vi "FPGA.vi"() -> ()   [LabVIEW 2020]
uses:
  <vilib>/Platform/TimedLoop/XDataNode/timing_clust.ctl
  <vilib>/Platform/TimedLoop/XDataNode/nitl_modes.ctl
  <vilib>/Platform/TimedLoop/XDataNode/wakeup.ctl
  <vilib>/rvi/Analysis/measure/FFT/simModelSupport/niFPGA FFT Sim Properties.ctl
  <vilib>/rvi/Analysis/measure/FFT/simModelSupport/niFPGA FFT Sim Types.ctl
  <vilib>/rvi/Analysis/measure/FFT/simModelSupport/niFpgaFFTSimArithmeticProperties.ctl
  <vilib>/rvi/Analysis/measure/FFT/simModelSupport/niFpgaFFTSimDfxp.ctl
  <vilib>/fxp/LVFixedPointQuantizationPolicyTypeDef.ctl
  <vilib>/rvi/eio/common/nirviEmuTemplateMethod_errors.vi
  <vilib>/rvi/DataTransferAndStorage/Container/Common/niFpgaContainerGetUniqueNameForEmu.vi
  <vilib>/rvi/DataTransferAndStorage/Container/Common/niFpgaContainerSetEmuInfo.vi
  <vilib>/rvi/eio/common/nirviEmuReportErrorAndStop.vi
  <vilib>/rvi/DataTransferAndStorage/Container/Common/niFpgaContainerExecOnDevCompGetState.vi
  <vilib>/rvi/Emulation/niFpgaEmulationIsFPGAContextNoSignature.vi
  <vilib>/rvi/Emulation/niFpgaSctlEmulationGetInTimedLoop.vi
  <vilib>/rvi/errors/niFpgaSetErrorForExecOnDevCompSimple.vi
  <vilib>/rvi/FIFO/Fifo_Resource/nirvififoEmulationSetSize.vi
  <vilib>/rvi/FIFO/Fifo_Resource/nirviFifoEmulationQueueMgr.vi
  <instcachedir>/0/nirviFifoEmulationQueueMgr_E5CAEC123FF24DC58D834DCA3CDAA9B5.lvgen/nirviFifoEmulationQueueMgr_E5CAEC123FF24DC58D834DCA3CDAA9B5_003.vi
  <vilib>/rvi/FIFO/Fifo_Resource/nirvififoEmulationDetermineInputValidOut.vi
  <vilib>/rvi/FIFO/Fifo_Resource/nirvififoEmulationCreateLock.vi
  <vilib>/rvi/Emulation/niFpgaProcessEmulError.vi
  <vilib>/rvi/FIFO/Fifo_Resource/nirvififoEmulationObtainLock.vi
  <vilib>/rvi/FIFO/Fifo_Resource/nirvififoEmulationReleaseLock.vi
  <vilib>/rvi/occurrence/nirviWaitOnOccurrenceBase.vi
  <vilib>/rvi/errors/nirviReportUnexpectedCaseInternalError.vi
  <vilib>/rvi/errors/nirviReportUnexpectedCaseInternalError (U32).vi
  <vilib>/Utility/error.llb/Clear Errors.vi
  <vilib>/rvi/interface/RandomDataEmulation/niFpgaRandomDataHandleErrors.vi
  <vilib>/rvi/Emulation/niFpgaEmulationReportErrorSimple.vi
  <vilib>/rvi/Emulation/niFpgaGetClockAttributes.vi
  <vilib>/rvi/Emulation/niFpgaCriticalErrorInLSC.vi
  <vilib>/rvi/Analysis/measure/FFT/simModelSupport/niFpgaFFTSimModelCore.vi
  <vilib>/eio/EIONode/EIONode.xnode
  <vilib>/rvi/LocalResourceManager/LocalResourceManager.xnode
  <vilib>/rvi/DataTransferAndStorage/Container/XNode/niFpgaContainer.xnode
  <vilib>/rvi/FIFO/Fifo_Resource/niFpgaFifoEmulationRefIn.vi
  <vilib>/Platform/TimedLoop/XDataNode/XDataNode.xnode
  <vilib>/rvi/interface/RandomDataEmulation/nirviRandomDataFpgaReadWriteTemplate.vi
  <vilib>/rvi/Analysis/measure/FFT/XNode/niFpgaFFT.xnode
  <vilib>/rvi/FXPMathLib/FxpInterpret/XNode/nifxpmath_Interpret.xnode
  <vilib>/Platform/TimedLoop/XDataNode/XDNodeRunTimeDep.lvlib
panel:
  out "Timed Out? FIFO out index 2":bool
  out "Timed Out? FIFO out IMG 2":bool
  out "Timed Out? FIFO out REAL 2":bool
  out "sort time (us)":u32
  out "Timed Out? FIFO in IMG":bool
  out "Timed Out? FIFO in REAL":bool
  out "Timed Out? FIFO out REAL":bool
  out "Timed Out? FIFO out IMG":bool
  out "Timed Out? FIFO out index":bool
  in  "FFT loop iterations":i32
  in  "auto stop":bool
  out "FFT time (uSec)":u32
  out "data collection time (uSec)":u32
  in  "Loop number":i32
  out "Element":fxp<+/-,24,7>
  out "Actual loop rate":u32
  in  "Rate (uSec)":u32 caption="Count(uSec)"
  out "Timed Out?":bool
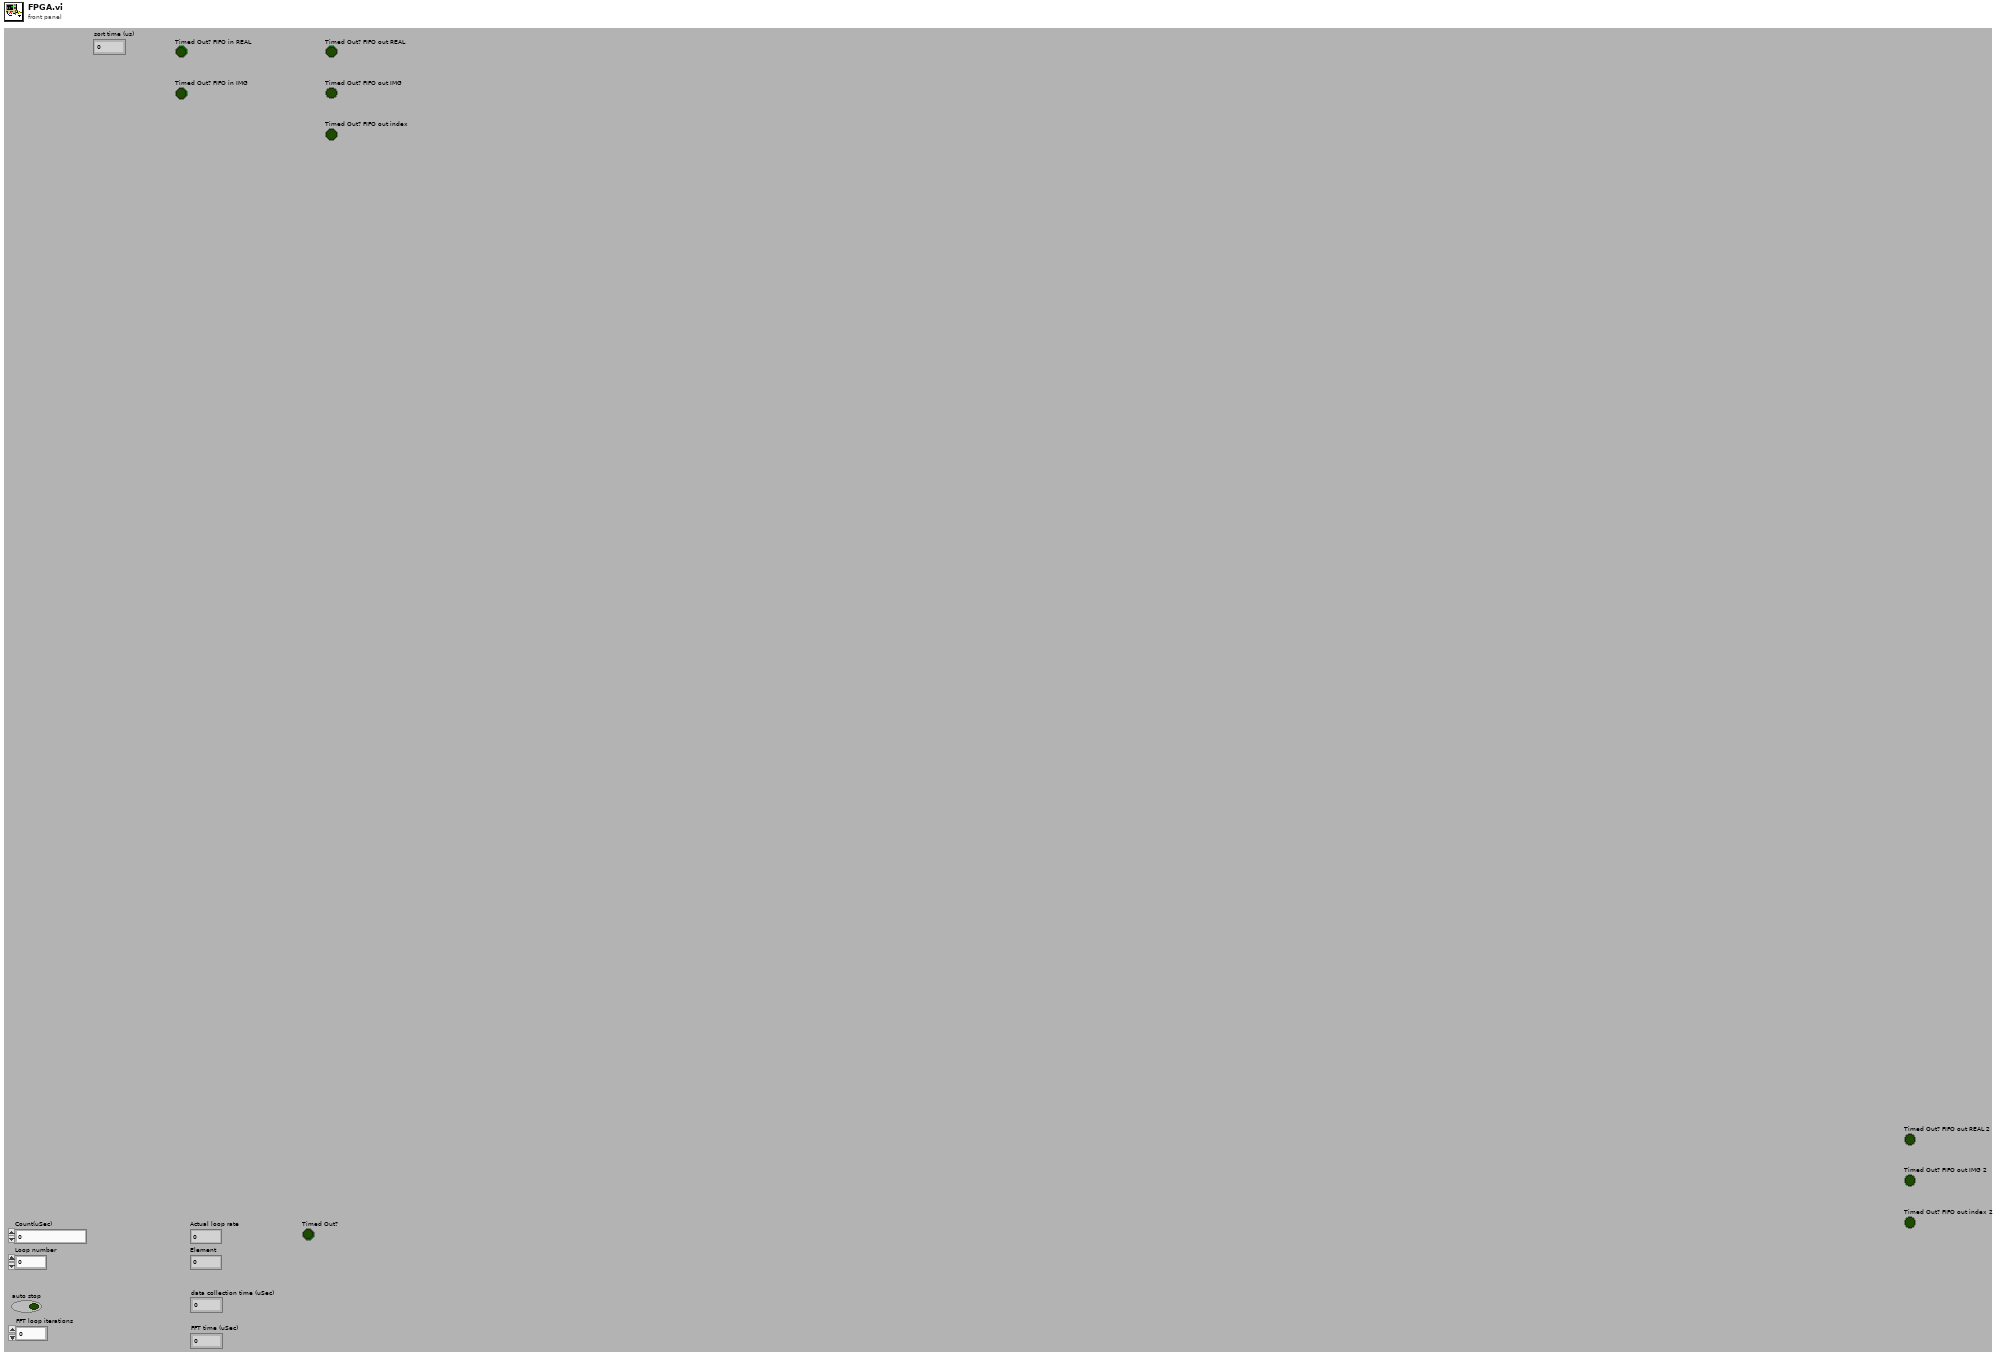
[diagram p1: front panel]
types:
  T1 = typedef "XDNodeRunTimeDep.lvlib/timing_clust.ctl" = cluster{"Expected End [f-1]":u64, "Actual End [f-1]":u64, "Finished Late? [f-1]":bool, "Expected End [i-1]":u64, "Actual End [i-1]":u64, "Finished Late? [i-1]":bool, "Expected Start [i]":u64, "Actual Start [i]":u64, "Expected Start [f]":u64, "Actual Start [f]":u64, "Source Name":string, "Structure Name":string, "Period":i64, "Deadline":i64, "Offset":i64, "Start":i64, "Priority":i32, "Timeout":i32, "Mode":T2, "Wakeup Reason":T3, "Error":errorcluster, "Source Type":string, "Secondary Source Type":string, "Global End Time":u64, "Global Start Time":u64, "Frame Duration":u64, "Iteration Duration":u64, "Assigned CPU":i32, "I/O Scan Engine Mode":u32}
  T2 = typedef "XDNodeRunTimeDep.lvlib/nitl_modes.ctl" = enum32{"No Change", "Process missed periods, maintain original phase", "Discard missed periods, maintain original phase", "Process missed periods, ignore original phase", "Discard missed periods, ignore original phase"}
  T3 = typedef "XDNodeRunTimeDep.lvlib/wakeup.ctl" = enum32{"Normal", "Aborted", "Asynchronous wakeup", "Timing source error", "Timed loop error", "Timeout"}
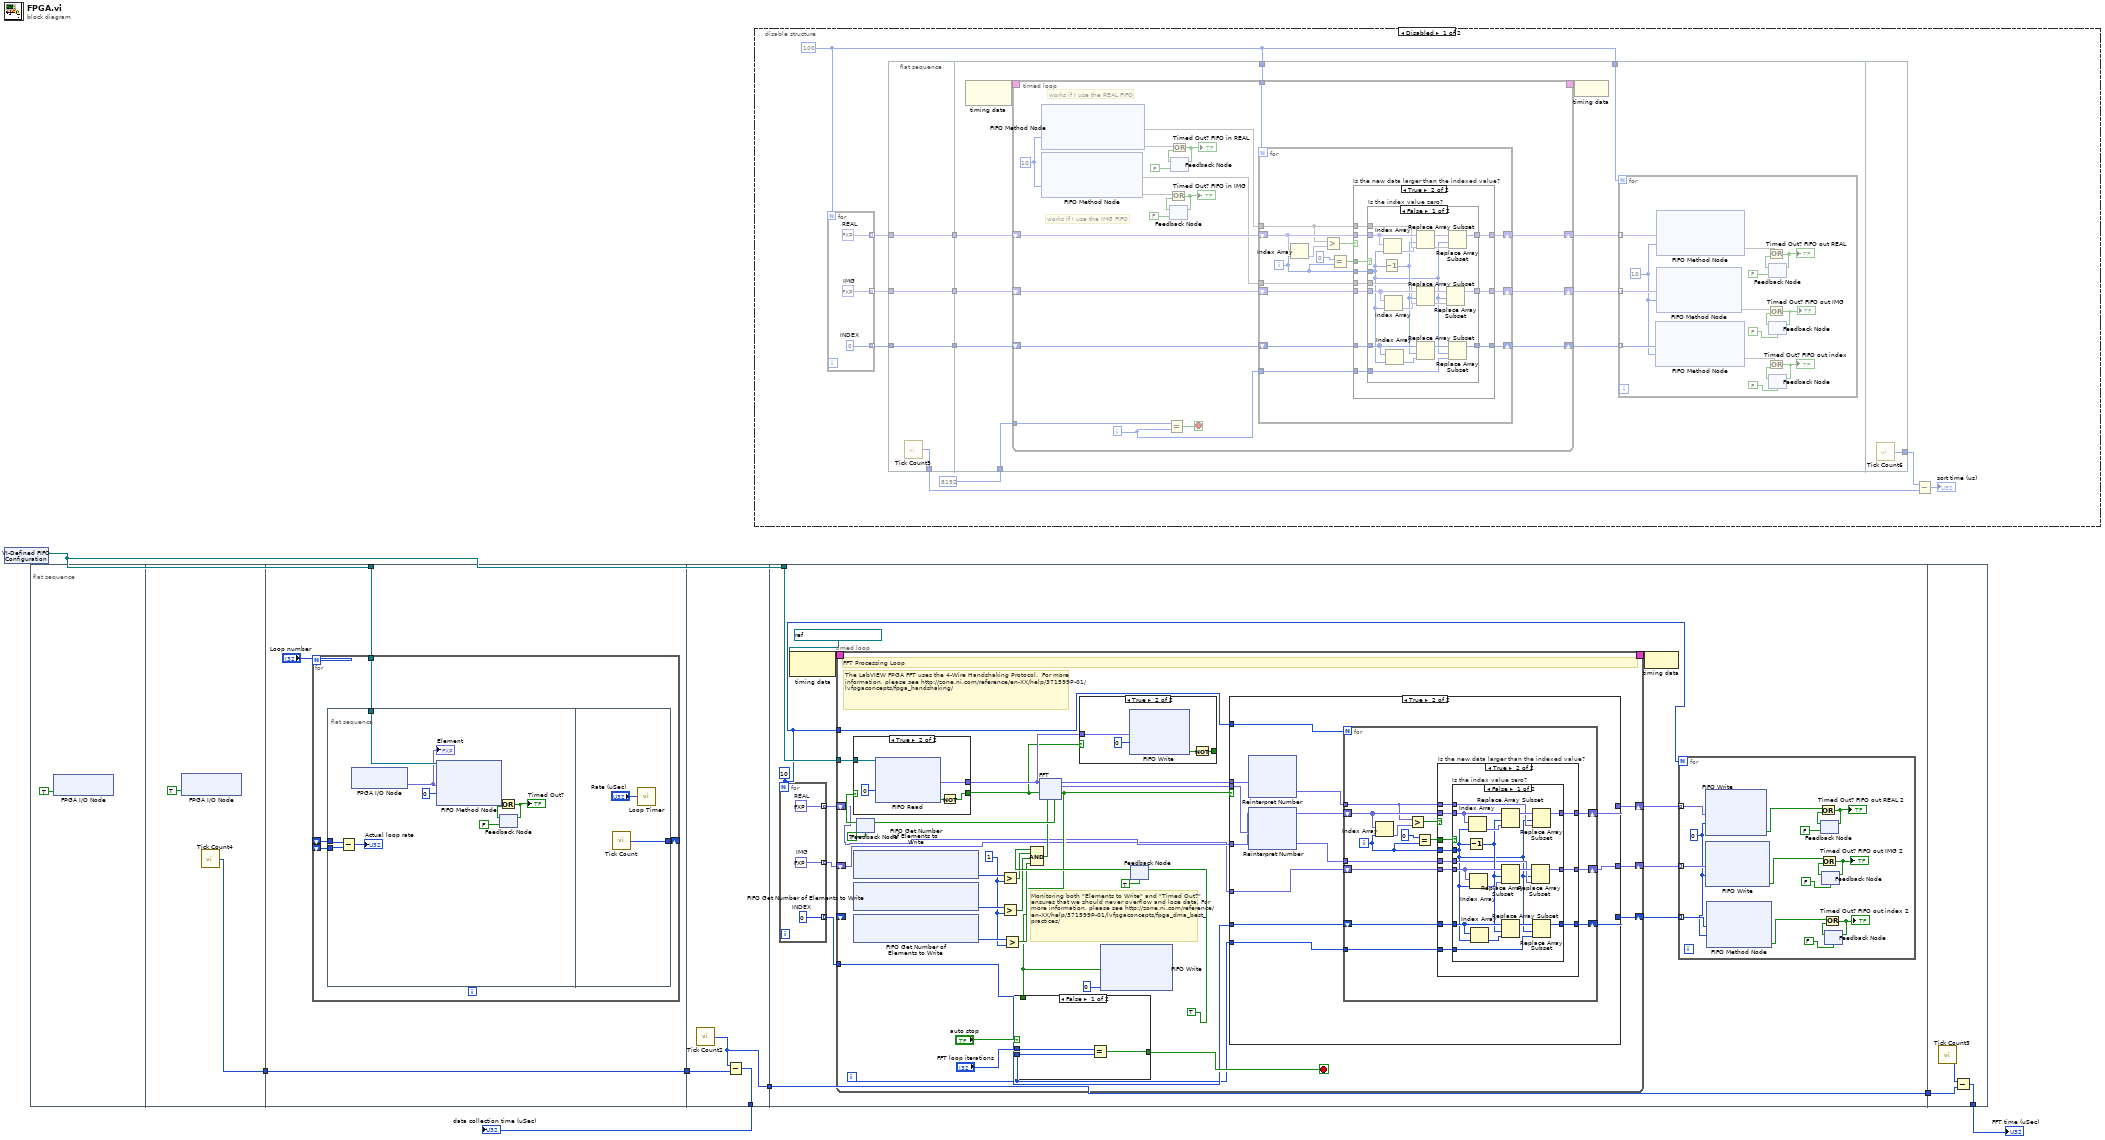
[diagram p0: block diagram]
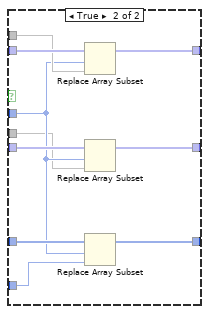
[diagram p3: hidden frame]
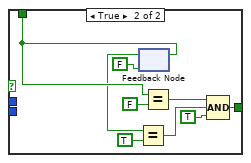
[diagram p5: hidden frame]
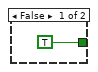
[diagram p6: hidden frame]
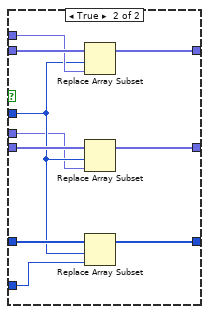
[diagram p9: hidden frame]
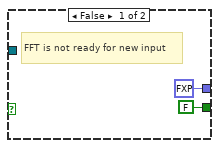
[diagram p10: hidden frame]
diagram:
  n1 = xnode "VI-Defined FIFO Configuration"() -> ("FIFO Out"=w7:refnum<k21>)
  n2 = flat-sequence {
    tunnel: [w9] -> w6
    tunnel: w7 -> [w13]
    tunnel: w6 -> [w11]
    tunnel: [w11] -> w5
    tunnel: w5 -> [w32]
    tunnel: [w31] -> w4
    tunnel: [w30] -> w3
    tunnel: w7 -> [w42]
    tunnel: w3 -> [w41]
    tunnel: [w41] -> w2
    tunnel: w2 -> [w223]
    tunnel: [w222] -> w1
    frame #0 {
      n3 = xnode "FPGA I/O Node"("Mod1/Stop"=TRUE) -> ()  [unwired: 1 in, 1 out]
    }
    frame #1 {
      n4 = xnode "FPGA I/O Node"("Mod1/Start"=TRUE) -> ()  [unwired: 1 in, 1 out]
      n5 = call "Tick Count4"() -> ("Tick Count(uSec)"=w9:u32)
    }
    frame #2 {
      n6 = for {
        N: "Loop number" -> [_]
        shift-right: [w17] -> _
        shift-left: _ -> [w16]
        shift-left: _ -> [w15]
        tunnel: w13 -> [w14]
        n7 = flat-sequence {
          tunnel: w16 -> [w27]
          tunnel: w15 -> [w26]
          tunnel: w14 -> [w19]
          tunnel: [w28] -> w17
          frame #0 {
            n8 = Subtract(x=w27, y=w26) -> (x-y=→"Actual loop rate":u32)
            n9 = xnode "FPGA I/O Node"() -> ("Mod1/AI0"=w18:fxp<+/-,24,7>)  [unwired: 1 in, 1 out]
            "Element" <- w18
            n10 = xnode ("FIFO Method Node")("Element"=w18, "Timeout"=0, "FIFO In"=w19) -> ("Timed Out?"=w23:bool)  [unwired: 1 in, 2 out]
            n11 = feedback #1(FALSE) -> (w22:bool)
            n12 = Or(x=w23, y=w22) -> (x .or. y?=w21:bool)
            "Timed Out?" <- w21
            n13 = feedback-in #1(w21) -> ()
          }
          frame #1 {
            n14 = call "Tick Count"() -> ("Tick Count(uSec)"=w28:u32)
            n15 = call "Loop Timer"("Count(uSec)"="Rate (uSec)") -> ()  [unwired: 1 out]
          }
        }
      }
    }
    frame #3 {
      n16 = call "Tick Count2"() -> ("Tick Count(uSec)"=w30:u32)
      n17 = Subtract(x=w30, y=w32) -> (x-y=w31:u32)
    }
    frame #4 {
      w34 = 10
      n18 = for {
        N: w34 -> [_]
        tunnel: [w63] -> w40 mode=indexing
        tunnel: [w62] -> w38 mode=indexing
        tunnel: [w61] -> w39 mode=indexing
        w61 = fxp<+/-,32,21> 0.0  # IMG
        w62 = 0  # INDEX
        w63 = fxp<+/-,32,21> 0.0  # REAL
      }
      n19 = node-c288(refnum<k21> "40 MHz Onboard Clock" ("Source Name")) -> (w44:T1)
      n20 = timed-loop {
        timing: w44 -> [_]
        timing-out: [_] -> w43
        tunnel: w42 -> [w92]
        tunnel: w38 -> [w70]
        tunnel: w34 -> [w64]
        shift-right: [w66] -> w35
        shift-left: _ -> [_]
        shift-right: [w67] -> w37
        shift-left: w39 -> [w71]
        shift-right: [w68] -> w36
        shift-left: w40 -> [w72]
        i -> [w69]
        stop <- w77 stop-if-true
        w86 = u32 1 ("y")
        # "Monitoring both \"Elements to Write\" and \"Timed Out?\" ensures that we should never overflow and lose data. For more information, please see http://zone.ni.com/reference/en-XX/help/371599P-01/lvfpgaconcepts/fpga_dma_best_practices/"
        # "The LabVIEW FPGA FFT uses the 4-Wire Handshaking Protocol.  For more information, please see http://zone.ni.com/reference/en-XX/help/371599P-01/lvfpgaconcepts/fpga_handshaking/"
        # "FFT Processing Loop"
        n21 = xnode ("FIFO Get Number of Elements to Write")() -> ("Number of Elements to Write"=w89:u32)  [unwired: 1 in, 1 out]
        n22 = xnode ("FIFO Get Number of Elements to Write")() -> ("Number of Elements to Write"=w88:u32)  [unwired: 1 in, 1 out]
        n23 = xnode ("FIFO Get Number of Elements to Write")() -> ("Number of Elements to Write"=w87:u32)  [unwired: 1 in, 1 out]
        n24 = feedback #2(TRUE ("ready for input")) -> (w95:bool)
        n25 = case shown="True" w95 {
          tunnel: [FALSE w214] -> w80
          tunnel: [fxp<+/-,16,5> 0.0 ("Element") w215] -> w94
          tunnel: w92 -> [_ w211]
          frame False {
            # "FFT is not ready for new input"
          }
          frame True {
            n26 = xnode ("FIFO Read")("Timeout"=0, "FIFO In"=w211) -> ("Element"=w215:fxp<+/-,24,7>, "Timed Out?"=w213:bool)  [unwired: 1 out]
            n27 = Not(x=w213) -> (.not. x?=w214:bool)
          }
        }
        n28 = Greater?(x=w89, y=w86) -> (0:w84:bool)
        n29 = Greater?(x=w88, y=w86) -> (0:w83:bool)
        n30 = Greater?(x=w87, y=w86) -> (0:w82:bool)
        n31 = case shown="True" w80 {
          tunnel: w94 -> [_ w109]
          tunnel: [TRUE ("Timed Out?") w110] -> _
          frame False {
          }
          frame True {
            n32 = xnode ("FIFO Write")("Element"=w109, "Timeout"=0) -> ("Timed Out?"=w111:bool)  [unwired: 1 in, 1 out]
            n33 = Not(x=w111) -> (.not. x?=w110:bool)
          }
        }
        n34 = feedback-in #3(TRUE) -> ()
        n35 = feedback #3(TRUE) -> (w85:bool)
        n36 = Compound Arithmetic op=AND(w85, w84, w83, w82) -> (w79:bool)
        n37 = xnode "FFT"("real data in"=w94, "input valid"=w80, "ready for output"=w79) -> ("ready for input"=w93:bool, "real data out"=w91:fxp<+/-,32,15>, "imaginary data out"=w76:fxp<+/-,32,15>, "output valid"=w73:bool)  [unwired: 2 in, 1 out]
        n38 = feedback-in #2(w93) -> ()
        n39 = case shown="False" "auto stop" {
          tunnel: w73 -> [_ w106]
          tunnel: [w96 w99] -> w77
          tunnel: w69 -> [w98 _]
          tunnel: "FFT loop iterations" -> [w97 _]
          frame False {
            n40 = Equal?(x=w97, y=w98) -> (x = y?=w96:bool)
          }
          frame True {
            n41 = feedback #4(FALSE) -> (w103:bool)
            n42 = Equal?(x=w103, y=TRUE) -> (x = y?=w101:bool)
            n43 = feedback-in #4(w106) -> ()
            n44 = Equal?(x=w106, y=FALSE) -> (x = y?=w102:bool)
            n45 = Compound Arithmetic op=AND(w102, w101, TRUE ("value")) -> (w99:bool)
          }
        }
        n46 = xnode ("FIFO Write")("Element"=w73, "Timeout"=0) -> ()  [unwired: 1 in, 2 out]
        n47 = case shown="True" w73 {
          tunnel: w91 -> [_ w153]
          tunnel: w76 -> [_ w152]
          tunnel: w72 -> [w141 w149]
          tunnel: w71 -> [w140 w148]
          tunnel: w70 -> [w139 w147]
          tunnel: w69 -> [_ w146]
          tunnel: [w141 w145] -> w68
          tunnel: [w140 w144] -> w67
          tunnel: [w139 w143] -> w66
          tunnel: w64 -> [_ w142]
          frame False {
          }
          frame True {
            n48 = xnode "Reinterpret Number"("x"=w153) -> ("y"=w151:fxp<+/-,32,21>)
            n49 = xnode "Reinterpret Number"("x"=w152) -> ("y"=w150:fxp<+/-,32,21>)
            n50 = for {
              N: w142 -> [_]
              tunnel: w151 -> [w164]
              shift-right: [w163] -> w145
              shift-left: w149 -> [w165]
              tunnel: w146 -> [w161]
              shift-right: [w159] -> w143
              shift-left: w147 -> [w160]
              shift-right: [w156] -> w144
              shift-left: w148 -> [w155]
              tunnel: w150 -> [w154]
              i -> [w162]
              n51 = Index Array(array=w165, index=w162) -> (element=w167:fxp<+/-,32,21>)
              n52 = Greater?(x=w164, y=w167) -> (0:w166:bool)
              n53 = Equal?(x=0, y=w162) -> (x = y?=w157:bool)
              n54 = case "Is the new data larger than the indexed value?" shown="True" w166 {
                tunnel: w165 -> [w170 w180]
                tunnel: w157 -> [_ w181]
                tunnel: w164 -> [_ w179]
                tunnel: w162 -> [_ w178]
                tunnel: [w170 w177] -> w163
                tunnel: w161 -> [_ w176]
                tunnel: w160 -> [w169 w175]
                tunnel: [w169 w174] -> w159
                tunnel: [w168 w173] -> w156
                tunnel: w155 -> [w168 w172]
                tunnel: w154 -> [_ w171]
                frame False {
                }
                frame True {
                  n55 = case "Is the index value zero?" shown="False" w181 {
                    tunnel: w180 -> [w198 w208]
                    tunnel: w179 -> [w195 w207]
                    tunnel: w178 -> [w182 w201]
                    tunnel: [w194 w206] -> w177
                    tunnel: w176 -> [w189 w205]
                    tunnel: w175 -> [w191 w204]
                    tunnel: [w190 w203] -> w174
                    tunnel: [w184 w199] -> w173
                    tunnel: w172 -> [w188 w202]
                    tunnel: w171 -> [w183 w200]
                    frame False {
                      n56 = Decrement(x=w182) -> (x-1=w186:i32)
                      n57 = Index Array(array=w198, index=w182) -> (element=w197:fxp<+/-,32,21>)
                      n58 = Index Array(array=w188, index=w182) -> (element=w187:fxp<+/-,32,21>)
                      n59 = Index Array(array=w191, index=w182) -> (element=w193:i32)
                      n60 = Replace Array Subset(array=w198, new element=w197, index=w186) -> (w196:fxp<+/-,32,21>[])
                      n61 = Replace Array Subset(array=w188, new element=w187, index=w186) -> (w185:fxp<+/-,32,21>[])
                      n62 = Replace Array Subset(array=w191, new element=w193, index=w186) -> (w192:i32[])
                      n63 = Replace Array Subset(array=w185, new element=w183, index=w182) -> (w184:fxp<+/-,32,21>[])
                      n64 = Replace Array Subset(array=w196, new element=w195, index=w182) -> (w194:fxp<+/-,32,21>[])
                      n65 = Replace Array Subset(array=w192, new element=w189, index=w182) -> (w190:i32[])
                    }
                    frame True {
                      n66 = Replace Array Subset(array=w208, new element=w207, index=w201) -> (w206:fxp<+/-,32,21>[])
                      n67 = Replace Array Subset(array=w202, new element=w200, index=w201) -> (w199:fxp<+/-,32,21>[])
                      n68 = Replace Array Subset(array=w204, new element=w205, index=w201) -> (w203:i32[])
                    }
                  }
                }
              }
            }
          }
        }
      }
      n69 = node-c288(w43) -> ()
      n70 = for {
        N: w34 -> [_]
        tunnel: w37 -> [w60] mode=indexing
        tunnel: w36 -> [w59] mode=indexing
        tunnel: w35 -> [w49] mode=indexing
        w48 = 0 ("Timeout")
        n71 = xnode ("FIFO Write")("Element"=w59, "Timeout"=w48) -> ("Timed Out?"=w45:bool)  [unwired: 1 in, 1 out]
        n72 = xnode ("FIFO Write")("Element"=w60, "Timeout"=w48) -> ("Timed Out?"=w46:bool)  [unwired: 1 in, 1 out]
        n73 = xnode ("FIFO Method Node")("Element"=w49, "Timeout"=w48) -> ("Timed Out?"=w47:bool)  [unwired: 1 in, 1 out]
        n74 = feedback #5(FALSE) -> (w56:bool)
        n75 = Or(x=w45, y=w56) -> (x .or. y?=w57:bool)
        "Timed Out? FIFO out REAL 2" <- w57
        n76 = feedback-in #5(w57) -> ()
        n77 = feedback #6(FALSE) -> (w55:bool)
        n78 = Or(x=w46, y=w55) -> (x .or. y?=w54:bool)
        "Timed Out? FIFO out IMG 2" <- w54
        n79 = feedback-in #6(w54) -> ()
        n80 = feedback #7(FALSE) -> (w52:bool)
        n81 = Or(x=w47, y=w52) -> (x .or. y?=w51:bool)
        "Timed Out? FIFO out index 2" <- w51
        n82 = feedback-in #7(w51) -> ()
      }
    }
    frame #5 {
      n83 = call "Tick Count3"() -> ("Tick Count(uSec)"=w224:u32)
      n84 = Subtract(x=w224, y=w223) -> (x-y=w222:u32)
    }
  }
  n85 = disable-structure shown="Disabled" {
    frame Disabled {
      w226 = 100
      n86 = for {
        N: w226 -> [_]
        tunnel: [w238] -> w228 mode=indexing
        tunnel: [w237] -> w229 mode=indexing
        tunnel: [w236] -> w225 mode=indexing
        w236 = fxp<+/-,32,21> 0.0  # IMG
        w237 = 0  # INDEX
        w238 = fxp<+/-,32,21> 0.0  # REAL
      }
      n87 = flat-sequence {
        tunnel: [w242] -> w231
        tunnel: [w241] -> w235
        tunnel: w229 -> [w241]
        tunnel: [w240] -> w234
        tunnel: w228 -> [w240]
        tunnel: [w239] -> w233
        tunnel: w225 -> [w239]
        tunnel: w235 -> [w253]
        tunnel: w234 -> [w252]
        tunnel: 8192 ("samples") -> [w250]
        tunnel: w226 -> [w251]
        tunnel: w226 -> [w247]
        tunnel: w233 -> [w243]
        tunnel: [w350] -> w232
        frame #0 {
          n88 = call "Tick Count5"() -> ("Tick Count(uSec)"=w242:u32)
        }
        frame #1 {
          n89 = node-c288() -> (w249:T1)  [unwired: 1 in]
          n90 = timed-loop {
            shift-right: [w289] -> w245
            shift-left: w252 -> [w290]
            shift-right: [w288] -> w246
            shift-left: w253 -> [w287]
            tunnel: w251 -> [w286]
            tunnel: w250 -> [w284]
            timing: w249 -> [_]
            timing-out: [_] -> w248
            shift-right: [w282] -> w244
            shift-left: w243 -> [w281]
            i -> [w285]
            stop <- w283 stop-if-true
            w280 = 10 ("Timeout")
            # "works if I use the REAL FIFO"
            # "works if I use the IMG FIFO"
            n91 = xnode ("FIFO Method Node")("Timeout"=w280) -> ("Element"=w278, "Timed Out?"=w270)  [unwired: 1 in, 1 out]
            n92 = xnode ("FIFO Method Node")("Timeout"=w280) -> ("Element"=w279, "Timed Out?"=w274)  [unwired: 1 in, 1 out]
            n93 = Equal?(x=w284, y=w285) -> (x = y?=w283:bool)
            n94 = feedback #8(FALSE) -> (w275:bool)
            n95 = Or(x=w274, y=w275) -> (x .or. y?=w276:bool)
            "Timed Out? FIFO in IMG" <- w276
            n96 = feedback-in #8(w276) -> ()
            n97 = feedback #9(FALSE) -> (w271:bool)
            n98 = Or(x=w270, y=w271) -> (x .or. y?=w272:bool)
            "Timed Out? FIFO in REAL" <- w272
            n99 = feedback-in #9(w272) -> ()
            n100 = for {
              N: w286 -> [_]
              tunnel: w278 -> [w301]
              shift-right: [w300] -> w289
              shift-left: w290 -> [w302]
              tunnel: w285 -> [w298]
              shift-right: [w296] -> w288
              shift-left: w287 -> [w297]
              shift-right: [w293] -> w282
              shift-left: w281 -> [w292]
              tunnel: w279 -> [w291]
              i -> [w299]
              n101 = Index Array(array=w302, index=w299) -> (element=w304:fxp<+/-,32,21>)
              n102 = Greater?(x=w301, y=w304) -> (0:w303:bool)
              n103 = Equal?(x=0, y=w299) -> (x = y?=w294:bool)
              n104 = case "Is the new data larger than the indexed value?" shown="True" w303 {
                tunnel: w302 -> [w307 w317]
                tunnel: w294 -> [_ w318]
                tunnel: w301 -> [_ w316]
                tunnel: w299 -> [_ w315]
                tunnel: [w307 w314] -> w300
                tunnel: w298 -> [_ w313]
                tunnel: w297 -> [w306 w312]
                tunnel: [w306 w311] -> w296
                tunnel: [w305 w310] -> w293
                tunnel: w292 -> [w305 w309]
                tunnel: w291 -> [_ w308]
                frame False {
                }
                frame True {
                  n105 = case "Is the index value zero?" shown="False" w318 {
                    tunnel: w317 -> [w335 w345]
                    tunnel: w316 -> [w332 w344]
                    tunnel: w315 -> [w319 w338]
                    tunnel: [w331 w343] -> w314
                    tunnel: w313 -> [w326 w342]
                    tunnel: w312 -> [w328 w341]
                    tunnel: [w327 w340] -> w311
                    tunnel: [w321 w336] -> w310
                    tunnel: w309 -> [w325 w339]
                    tunnel: w308 -> [w320 w337]
                    frame False {
                      n106 = Decrement(x=w319) -> (x-1=w323:i32)
                      n107 = Index Array(array=w335, index=w319) -> (element=w334:fxp<+/-,32,21>)
                      n108 = Index Array(array=w325, index=w319) -> (element=w324:fxp<+/-,32,21>)
                      n109 = Index Array(array=w328, index=w319) -> (element=w330:i32)
                      n110 = Replace Array Subset(array=w335, new element=w334, index=w323) -> (w333:fxp<+/-,32,21>[])
                      n111 = Replace Array Subset(array=w325, new element=w324, index=w323) -> (w322:fxp<+/-,32,21>[])
                      n112 = Replace Array Subset(array=w328, new element=w330, index=w323) -> (w329:i32[])
                      n113 = Replace Array Subset(array=w322, new element=w320, index=w319) -> (w321:fxp<+/-,32,21>[])
                      n114 = Replace Array Subset(array=w333, new element=w332, index=w319) -> (w331:fxp<+/-,32,21>[])
                      n115 = Replace Array Subset(array=w329, new element=w326, index=w319) -> (w327:i32[])
                    }
                    frame True {
                      n116 = Replace Array Subset(array=w345, new element=w344, index=w338) -> (w343:fxp<+/-,32,21>[])
                      n117 = Replace Array Subset(array=w339, new element=w337, index=w338) -> (w336:fxp<+/-,32,21>[])
                      n118 = Replace Array Subset(array=w341, new element=w342, index=w338) -> (w340:i32[])
                    }
                  }
                }
              }
            }
          }
          n119 = node-c288(w248) -> ()
          n120 = for {
            N: w247 -> [_]
            tunnel: w246 -> [w269] mode=indexing
            tunnel: w245 -> [w268] mode=indexing
            tunnel: w244 -> [w267] mode=indexing
            w266 = 10 ("Timeout")
            n121 = xnode ("FIFO Method Node")("Element"=w269, "Timeout"=w266) -> ("Timed Out?"=w254)  [unwired: 1 in, 1 out]
            n122 = xnode ("FIFO Method Node")("Element"=w268, "Timeout"=w266) -> ("Timed Out?"=w262)  [unwired: 1 in, 1 out]
            n123 = xnode ("FIFO Method Node")("Element"=w267, "Timeout"=w266) -> ("Timed Out?"=w258)  [unwired: 1 in, 1 out]
            n124 = feedback #10(FALSE) -> (w263:bool)
            n125 = Or(x=w262, y=w263) -> (x .or. y?=w264:bool)
            "Timed Out? FIFO out REAL" <- w264
            n126 = feedback-in #10(w264) -> ()
            n127 = feedback #11(FALSE) -> (w261:bool)
            n128 = Or(x=w258, y=w261) -> (x .or. y?=w260:bool)
            "Timed Out? FIFO out IMG" <- w260
            n129 = feedback-in #11(w260) -> ()
            n130 = feedback #12(FALSE) -> (w257:bool)
            n131 = Or(x=w254, y=w257) -> (x .or. y?=w256:bool)
            "Timed Out? FIFO out index" <- w256
            n132 = feedback-in #12(w256) -> ()
          }
        }
        frame #2 {
          n133 = call "Tick Count6"() -> ("Tick Count(uSec)"=w350:u32)
        }
      }
      n134 = Subtract(x=w232, y=w231) -> (x-y=→"sort time (us)":u32)
    }
    frame Enabled {
    }
  }
  "data collection time (uSec)" <- w4
  "FFT time (uSec)" <- w1
